vi "Load_experiment.vi"(8 "error in (no error)":errorcluster, 11 "XML Elements":string) -> (0 "error IO":errorcluster, 3 "Experiment parameters":T1={"Stimulus signal"={"Effector"="On-screen signal", "Delay"=-100.0}, "Reward period signal"={"Effector"="On-screen signal", "Delay"=0.0}, "Reward"={"Effector"="On-screen signal", "Condition"="In window", "Delay"=100.0}, "Response"={"Source"="Keyboard", "Window start"=0.0, "Threshold"=1, "Window duration"=250.0}, "Punishment"={"Effector"="On-screen signal", "Condition"="Wrong response"}})   [LabVIEW 2016]
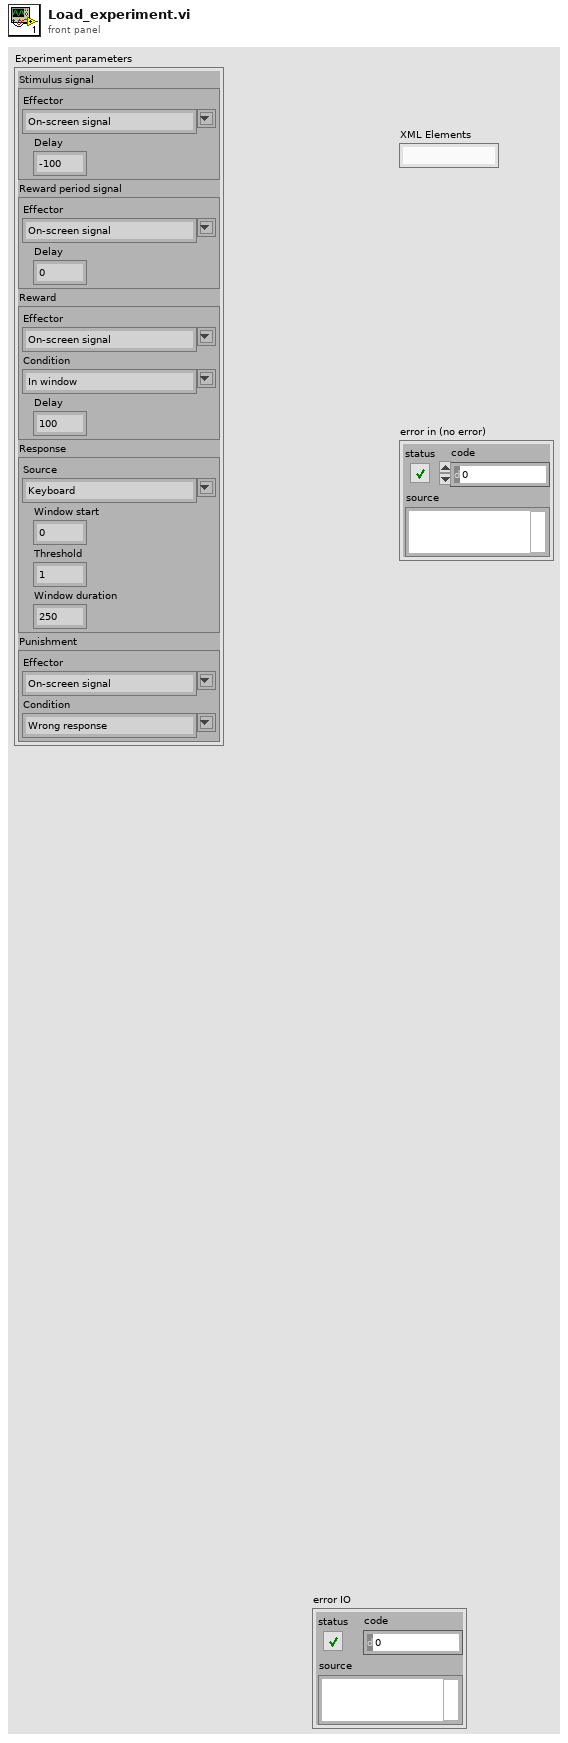
[diagram p1: front panel]
types:
  T1 = cluster{"Stimulus signal":cluster{"Effector":string, "Delay":dbl}, "Reward period signal":cluster{"Effector":string, "Delay":dbl}, "Reward":cluster{"Effector":string, "Condition":string, "Delay":dbl}, "Response":cluster{"Source":string, "Window start":dbl, "Threshold":u32, "Window duration":dbl}, "Punishment":cluster{"Effector":string, "Condition":string}}
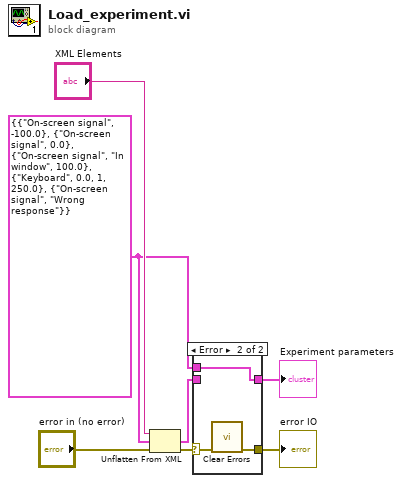
[diagram p0: block diagram]
diagram:
  w2 = T1 {"Stimulus signal"={"Effector"="On-screen signal", "Delay"=-100.0}, "Reward period signal"={"Effector"="On-screen signal", "Delay"=0.0}, "Reward"={"Effector"="On-screen signal", "Condition"="In window", "Delay"=100.0}, "Response"={"Source"="Keyboard", "Window start"=0.0, "Threshold"=1, "Window duration"=250.0}, "Punishment"={"Effector"="On-screen signal", "Condition"="Wrong response"}} ("Experiment parameters")
  n1 = Unflatten From XML(xml string="XML Elements", type=w2, error in (no error)="error in (no error)") -> (value=w3:T1, error out=w5:errorcluster)
  n2 = case shown="Error" w5 {
    selector: w5 -> [w9 w12]
    tunnel: [w9 w11] -> w4
    tunnel: [w8 w10] -> w1
    tunnel: w3 -> [w8 _]
    tunnel: w2 -> [_ w10]
    frame No Error {
    }
    frame Error {
      n3 = call <vilib>:"Clear Errors.vi"("error in (no error)"=w12) -> ("error out"=w11:errorcluster)  [unwired: 5 in, 1 out]
    }
  }
  "error IO" <- w4
  "Experiment parameters" <- w1
